vi "Stepper Sequence.vi"() -> ()   [LabVIEW 2013, in "LabVIEW Interface for Arduino.lvlib"]
doc: "Writes specified digital values to all 14 digital I/O pins. Each pin must first be configured as a digital output using the Arduino Set Digital Pin Mode VI."
uses:
  <vilib>/LabVIEW Interface for Arduino/LabVIEW Interface for Arduino.lvlib
  Hello Optotune Lens (30.06.2014)/Calibration.ctl
  <vilib>/LabVIEW Interface for Arduino/Type Defs/Board Type.ctl
  <vilib>/LabVIEW Interface for Arduino/Type Defs/Analog Pin.ctl
  <vilib>/Instr/_visa.llb/VISA Configure Serial Port (Instr).vi
panel:
  out "Array":dbl[](array[numeric])
  out "Voltage":dbl(knob) scale=0.0..5.0
  out "x*y 2":dbl
  out "x*y":dbl
  out "8bit integer":i8
  out "Schritt 7":bool=TRUE
  out "Schritt 6":bool=TRUE
  out "Schritt 5":bool=TRUE
  out "Schritt 4":bool=TRUE
  out "Schritt 3":bool=TRUE
  out "Schritt 2":bool=TRUE
  out "Schritt 1":bool=TRUE
  out "Value":u8
  out "x = y?":bool
  in  "Threshold I_Focus":dbl=0.33
  out "Nummer Aktuelle Messung":i32
  out "Position_aktuell 2":dbl
  out "Result":dbl[][](array[numeric])
  out "x+y":dbl
  in  "STOP Process":bool
  in  "STOP INTIAL":bool
  out "VISA resource name out 3":refnum<visa-resource-name>
  out "Command to Port 2":string
  out "Number of Measurements":i8
  in  "Min Focal Length 2":dbl
  in  "Max Focal Length":dbl=293.0
  out "I_0 - I_aktuell":dbl
  out "I_new":dbl(knob) scale=0.0..5.0
  out "Steps":dbl
  out "Position_aktuell":dbl
  in  "First Motor Pin":u8=3
  in  "Pin Endlagenschalter":u8=32
  out "I_0":dbl(knob) scale=0.0..5.0
  in  "Stepwidth Focalwidth lens":dbl=50.0
  in  "Calibration":T1={"Max Current A"=293.0, "Max Current B"=293.0, "UCL A"=300.0, "UCL B"=300.0, "LCL A"=0.0, "LCL B"=0.0} {"Max Current A" format="%#_g mA"; "Max Current B" format="%#_g mA"; "UCL A" format="%#_g mA"; "LCL A" format="%#_g mA"; "UCL B" format="%#_g mA"; "LCL B" format="%#_g mA"}
  out "ID":u16
  out "VISA resource name out":string
  out "Calibration 2":T1 {"Max Current A" format="%#_g mA"; "Max Current B" format="%#_g mA"; "UCL A" format="%#_g mA"; "LCL A" format="%#_g mA"; "UCL B" format="%#_g mA"; "LCL B" format="%#_g mA"}
  out "OK":bool
  out "Data":string
  out "Command to Port":string
  out "TA (°C)":dbl
  out "error out":errorcluster
  in  "error in (no error)":errorcluster
  in  "VISA resource name":string="COM13"
  in  "Initial Speed":dbl=1.0
  # "Lens Settings"
  # "Diodenstrom I0"
  # "Measurement Settings"
  # "Initial Settings"
  # "mA"
  # "0 Fast, 100 slow"
  # "mA"
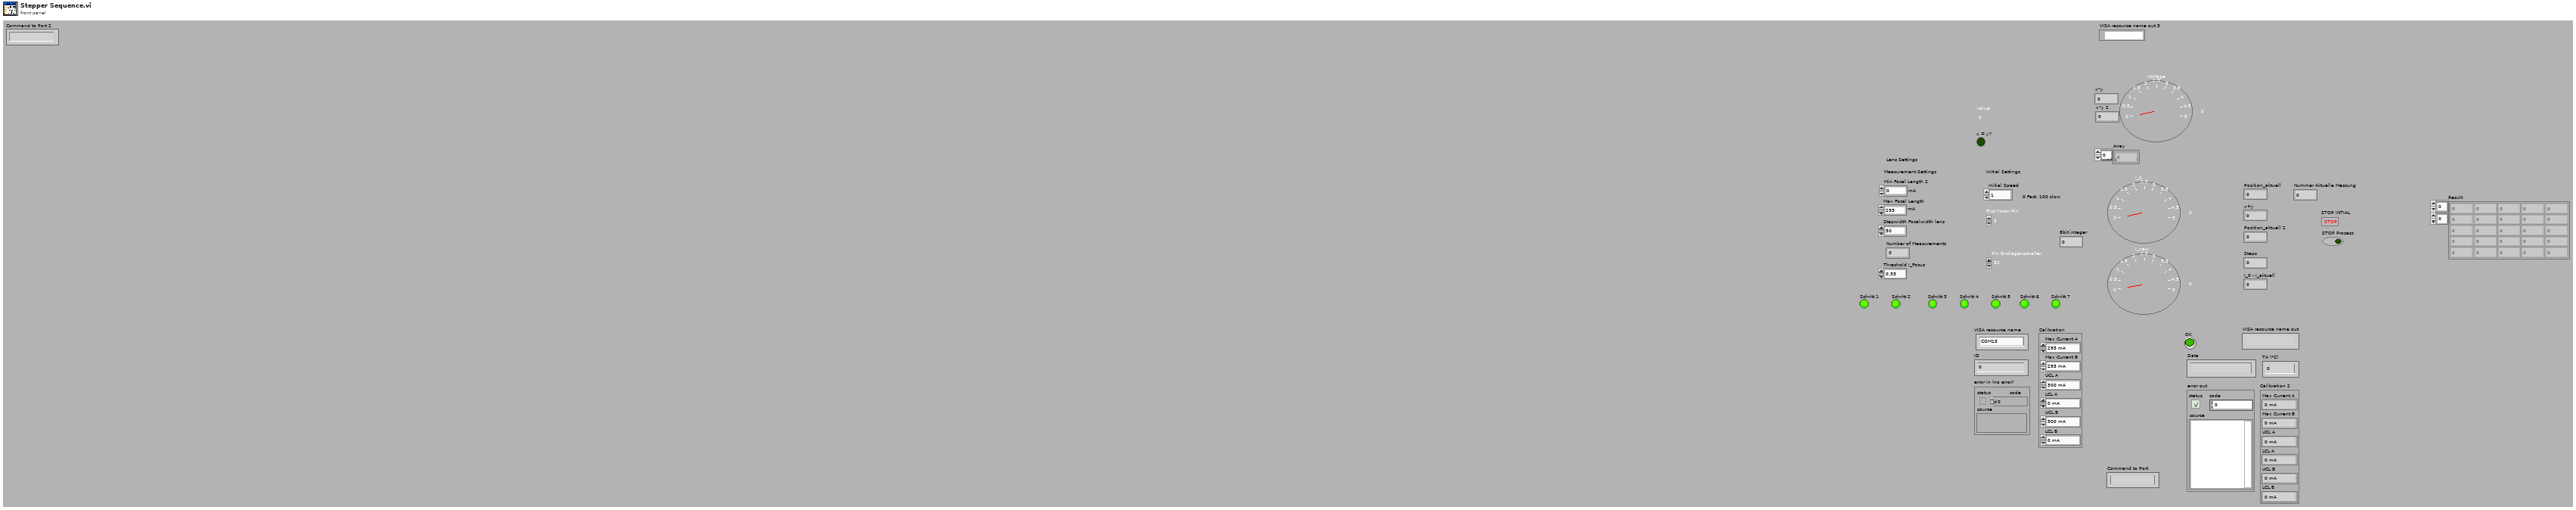
[diagram p1: front panel]
types:
  T1 = typedef "Calibration.ctl" = cluster{"Max Current A":dbl, "Max Current B":dbl, "UCL A":dbl, "UCL B":dbl, "LCL A":dbl, "LCL B":dbl}
  T2 = typedef "LabVIEW Interface for Arduino.lvlib/Board Type.ctl" = enum16{"Uno", "Dimuelanove w/Atmega 328", "Mega 2560"}
  T3 = typedef "LabVIEW Interface for Arduino.lvlib/Arduino Resource.ctl" = cluster{"VISA resource":refnum<visa-resource-name>, "Board Type":T2, "Connection Type":enum8{"USB / Serial"}, "Bytes Per Packet (15)":u8}
  T4 = typedef "LabVIEW Interface for Arduino.lvlib/Analog Pin.ctl" = enum8{"Anlog In 0", "Anlog In 1", "Anlog In 2", "Anlog In 3", "Anlog In 4", "Anlog In 5"}
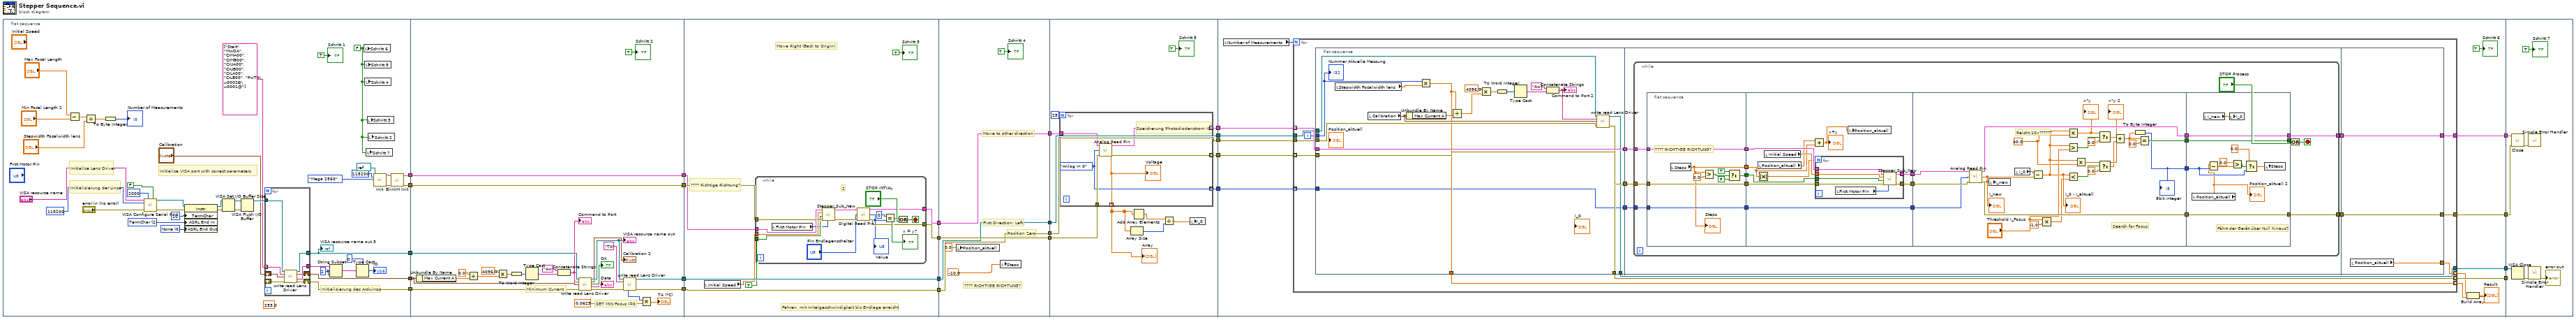
[diagram p0: block diagram]
diagram:
  n1 = flat-sequence {
    tunnel: [w44] -> w16
    tunnel: [w43] -> w15
    tunnel: [w42] -> w14
    tunnel: [w37] -> w3
    tunnel: [w36] -> w2
    tunnel: [w78] -> w26
    tunnel: [w77] -> w25
    tunnel: w16 -> [w100]
    tunnel: w15 -> [w99]
    tunnel: w14 -> [w98]
    tunnel: [w95] -> w13
    tunnel: [w79] -> w4
    tunnel: w3 -> [w78]
    tunnel: w2 -> [w77]
    tunnel: [w108] -> w20
    tunnel: w26 -> [w106]
    tunnel: [w107] -> w18
    tunnel: w25 -> [w109]
    tunnel: w13 -> [w105]
    tunnel: [w105] -> w12
    tunnel: [w104] -> w5
    tunnel: w4 -> [w104]
    tunnel: w20 -> [w131]
    tunnel: [w131] -> w19
    tunnel: w18 -> [w130]
    tunnel: [w130] -> w17
    tunnel: w12 -> [w129]
    tunnel: [w129] -> w11
    tunnel: [w128] -> w6
    tunnel: w5 -> [w128]
    tunnel: w19 -> [w143]
    tunnel: [w142] -> w24
    tunnel: w17 -> [w144]
    tunnel: [w141] -> w23
    tunnel: w11 -> [w140]
    tunnel: [w140] -> w10
    tunnel: [w139] -> w7
    tunnel: w6 -> [w139]
    tunnel: [w138] -> w1
    tunnel: w24 -> [w164]
    tunnel: w23 -> [w163]
    tunnel: [w162] -> w22
    tunnel: [w161] -> w21
    tunnel: w10 -> [w158]
    tunnel: [w159] -> w9
    tunnel: [w157] -> w8
    tunnel: w7 -> [w156]
    tunnel: w1 -> [w152]
    tunnel: w22 -> [w293]
    tunnel: w21 -> [w292]
    tunnel: w9 -> [w294]
    tunnel: w8 -> [_]
    frame #0 {
      w28 = FALSE ("Schritt 6")
      (unwired) 293.0
      w64 = 2 ("length (rest)")
      w49 = u16 0 items=["None", "Last Bit", "TermChar", "Break"] ("Serial Settings:End Mode for Writes")
      w50 = u16 2 items=["None", "Last Bit", "TermChar"] ("Serial Settings:End Mode for Reads")
      # "Initialisierung des Arduinos"
      # "Initialisierung der Linse"
      # "Initialize Lens Driver"
      # "Initialize VISA port with correct parameters"
      n2 = Subtract(x="Max Focal Length", y="Min Focal Length 2") -> (x-y=w33:dbl)
      n3 = Divide(x=w33, y="Stepwidth Focalwidth lens") -> (x/y=w31:dbl)
      n4 = To Byte Integer(number=w31) -> (8bit integer=→"Number of Measurements":i8)
      n5 = call-poly "VISA Configure Serial Port"("VISA resource name"="VISA resource name", "timeout (10sec)"=u32 2000, "Enable Termination\nChar (T)"=FALSE ("Enable Termination\nChar (T)"), "baud rate (9600)"=u32 115200, "error in (no error)"="error in (no error)") -> ("VISA resource name out"=w54:refnum<visa-resource-name>, "error out"=w52:errorcluster)  [unwired: 9 in]
      n6 = property class="Instr"(reference=w54, error in=w52, "TermChar"=u8 10 ("Message Based Settings:Termination Character"), "ASRL End In"=w50, "ASRL End Out"=w49) -> (reference out=w53:refnum<visa-resource-name>, error out=w51:errorcluster)
      n7 = VISA Set I/O Buffer Size(VISA resource name=w53, error in (no error)=w51) -> (VISA resource name out=w46:refnum<visa-resource-name>, error out=w45:errorcluster)  [unwired: 2 in]
      n8 = VISA Flush I/O Buffer(VISA resource name=w46, error in (no error)=w45) -> (VISA resource name out=w66:refnum<visa-resource-name>)  [unwired: 1 in, 1 out]
      n9 = for {
        tunnel: w66 -> [w73]
        tunnel: [w70] -> w44
        tunnel: string[] ["Start", "MwDA", "CrMA00", "CrMB00", "CrUA00", "CrUB00", "CrLA00", "CrLB00", "PwTA\u0002Ð\u0001@"] -> [w68] mode=indexing
        tunnel: [w67] -> w60
        shift-right: [w71] -> w43
        shift-left: "Calibration" -> [w72]
        shift-right: [w69] -> w42
        shift-left: _ -> [w74]
        n10 = call "write read Lens Driver.vi"("VISA resource name"=w73, "command"=w68, "Calibration"=w72, "error in (no error)"=w74) -> ("VISA resource name out"=w70:refnum<visa-resource-name>, "Calibration 2"=w71:T1, "Data"=w67:string, "error out"=w69:errorcluster)  [unwired: 4 in, 4 out]
      }
      "VISA resource name out 3" <- w44
      n11 = String Subset(string=w60, offset (0)=w64, length (rest)=w64) -> (substring=w62:string)
      n12 = Type Cast(type=u16 0 ("length (rest)"), x=w62) -> (*(type *) &x=→"ID":u16)
      n13 = local write "Schritt 6"(w28) -> ()
      n14 = local write "Schritt 5"(w28) -> ()
      n15 = local write "Schritt 4"(w28) -> ()
      n16 = local write "Schritt 7"(w28) -> ()
      n17 = local write "Schritt 3"(w28) -> ()
      n18 = local write "Schritt 2"(w28) -> ()
      n19 = call <vilib>:"Init.vi"("VISA resource"=refnum<visa-resource-name> refnum, "Baud Rate (115200)"=u32 115200, "Board Type (Uno)"=Board_Type."Mega 2560") -> ("Arduino Resource"=w40:T3, "error out"=w41:errorcluster)  [unwired: 15 in]
      n20 = call <vilib>:"BlinkM Init.vi"("Arduino Resource"=w40, "error in"=w41) -> ("Arduino Resource"=w37:T3, "error out"=w36:errorcluster)  [unwired: 12 in]
      "Schritt 1" <- TRUE
    }
    frame #1 {
      # "Minimum Current"
      # "SET MIN Focus I=0"
      n21 = Unbundle By Name(w99) -> ("Max Current A"=w84:dbl)
      n22 = Divide(x=0.0, y=w84) -> (x/y=w91:dbl)
      n23 = Multiply(x=4096.0, y=w91) -> (x*y=w89:dbl)
      n24 = To Word Integer(number=w89) -> (16bit integer=w88:i16)
      n25 = Type Cast(x=w88) -> (*(type *) &x=w87:string)  [unwired: 1 in]
      n26 = Concatenate Strings("Aw", w87) -> (w85:string)
      "Command to Port" <- w85
      n27 = call "write read Lens Driver.vi"("VISA resource name"=w100, "command"=w85, "Calibration"=w99, "error in (no error)"=w98) -> ("VISA resource name out"=w97:refnum<visa-resource-name>, "Calibration 2"=→"Calibration 2":T1, "OK"=→"OK":bool, "Data"=→"Data":string, "error out"=w96:errorcluster)  [unwired: 4 in, 3 out]
      "VISA resource name out" <- w97
      n28 = call "write read Lens Driver.vi"("VISA resource name"=w97, "command"="TA", "error in (no error)"=w96) -> ("VISA resource name out"=w95:refnum<visa-resource-name>, "TA"=w81:u16, "error out"=w79:errorcluster)  [unwired: 5 in, 5 out]
      n29 = Multiply(x=w81, y=0.0625) -> (x*y=→"TA (°C)":dbl)
      "Schritt 2" <- TRUE
    }
    frame #2 {
      # "???? Richtige Richtung?"
      # "Move Right (Back to Origin)"
      # "Fahren, mit Initalgeschwindigkeit bis Endlage erreicht"
      n30 = local read "Initial Speed"() -> (w103:dbl)
      n31 = while {
        tunnel: w106 -> [w123]
        tunnel: w109 -> [w122]
        tunnel: TRUE -> [w120]
        tunnel: w103 -> [w121]
        tunnel: [w115] -> w108
        tunnel: [w114] -> w107
        stop <- w117 stop-if-true
        # "2"
        n32 = local read "First Motor Pin"() -> (w119:u8)
        n33 = call "Stepper_Sub_New.vi"("First Motor Pin"=w119, "error in"=w122, "Direction"=w120, "Velocity"=w121, "Arduino Resource"=w123) -> ("error out"=w112:errorcluster, "Arduino Resource 2"=w111:T3)  [unwired: 5 in]
        n34 = call <vilib>:"Digital Read Pin.vi"("Arduino Resource"=w111, "Digital I/O Pin (0)"="Pin Endlagenschalter", "error in"=w112) -> ("Arduino Resource"=w115:T3, "Value"=w113:u8, "error out"=w114:errorcluster)  [unwired: 10 in]
        "Value" <- w113
        n35 = Equal?(x=u8 0, y=w113) -> (x = y?=w118:bool)
        "x = y?" <- w118
        n36 = Or(x=w118, y="STOP INTIAL") -> (x .or. y?=w117:bool)
      }
      "Schritt 3" <- TRUE
    }
    frame #3 {
      # "???? RICHTIGE RICHTUNG?"
      # "Move to other direction"
      # "First Direction: Left"
      # "Position Zero"
      n37 = local write "Position_aktuell"(0.0 ("Position_aktuell")) -> ()
      n38 = local write "Steps"(-10.0 ("Position_aktuell")) -> ()
      "Schritt 4" <- TRUE
    }
    frame #4 {
      n39 = for {
        N: 25 -> [_]
        tunnel: w144 -> [w150]
        tunnel: w143 -> [w149]
        tunnel: [w148] -> w142 mode=indexing
        tunnel: [w147] -> w141 mode=indexing
        tunnel: [w146] -> w138 mode=indexing
        tunnel: [w145] -> w136 mode=indexing
        w146 = Analog_Pin."Anlog In 0" ("Photodiode Pin")
        # "Speicherung Photodiodenstrom I0"
        n40 = call <vilib>:"Analog Read Pin.vi"("Arduino Resource"=w149, "Analog Input Pin (0)"=w146, "error in"=w150) -> ("Arduino Resource"=w148:T3, "Voltage"=w145:dbl, "error out"=w147:errorcluster)  [unwired: 10 in]
        "Voltage" <- w145
      }
      "Array" <- w136
      n41 = Array Size(array=w136) -> (size(s)=w134:i32)
      n42 = Add Array Elements(numeric array=w136) -> (sum=w135:dbl)
      n43 = Divide(x=w135, y=w134) -> (x/y=w133:dbl)
      n44 = local write "I_0"(w133) -> ()
      "Schritt 5" <- TRUE
    }
    frame #5 {
      n45 = local read "Number of Measurements"() -> (w160:i8)
      n46 = for {
        N: w160 -> [_]
        tunnel: w164 -> [w181] mode=indexing
        tunnel: w163 -> [w180] mode=indexing
        tunnel: [w179] -> w162
        tunnel: [w178] -> w161
        tunnel: w158 -> [w175]
        tunnel: w156 -> [w174]
        tunnel: [w172] -> w159
        tunnel: [w171] -> w157 mode=indexing
        tunnel: [w168] -> w155 mode=indexing
        tunnel: [w167] -> w154 mode=indexing
        tunnel: w152 -> [w165] mode=indexing
        i -> [w173]
        n47 = flat-sequence {
          tunnel: w181 -> [w200]
          tunnel: [w200] -> w177
          tunnel: w180 -> [w199]
          tunnel: [w199] -> w176
          tunnel: w175 -> [w191]
          tunnel: w174 -> [w190]
          tunnel: w173 -> [w187]
          tunnel: [w186] -> w172
          tunnel: [w185] -> w171
          tunnel: [w183] -> w167
          tunnel: [w182] -> w166
          tunnel: w165 -> [w182]
          tunnel: w177 -> [w205]
          tunnel: w176 -> [w204]
          tunnel: [w203] -> w170
          tunnel: [w202] -> w169
          tunnel: w166 -> [w201]
          tunnel: [w289] -> w178
          tunnel: [w290] -> w179
          tunnel: w170 -> [w290]
          tunnel: w169 -> [w289]
          tunnel: [w288] -> w168
          frame #0 {
            n48 = local read "Stepwidth Focalwidth lens"() -> (w188:dbl)
            n49 = local read "Calibration"() -> (w184:T1)
            n50 = Unbundle By Name(w184) -> ("Max Current A"=w189:dbl)
            n51 = Multiply(x=w187, y=w188) -> (x*y=w183:dbl)
            n52 = Divide(x=w183, y=w189) -> (x/y=w198:dbl)
            n53 = Multiply(x=4096.0, y=w198) -> (x*y=w196:dbl)
            n54 = To Word Integer(number=w196) -> (16bit integer=w195:i16)
            n55 = Type Cast(x=w195) -> (*(type *) &x=w194:string)  [unwired: 1 in]
            n56 = Concatenate Strings("Aw", w194) -> (w192:string)
            "Command to Port 2" <- w192
            n57 = call "write read Lens Driver.vi"("VISA resource name"=w191, "command"=w192, "Calibration"=w184, "error in (no error)"=w190) -> ("VISA resource name out"=w186:refnum<visa-resource-name>, "error out"=w185:errorcluster)  [unwired: 4 in, 6 out]
            "Nummer Aktuelle Messung" <- w187
          }
          frame #1 {
            n58 = while {
              tunnel: w205 -> [w223]
              tunnel: w204 -> [w222]
              tunnel: [w221] -> w203
              tunnel: [w220] -> w202
              tunnel: w201 -> [w207]
              stop <- w218 stop-if-true
              n59 = flat-sequence {
                tunnel: w222 -> [w233]
                tunnel: w223 -> [w234]
                tunnel: [w234] -> w214
                tunnel: [w233] -> w213
                tunnel: [w226] -> w212
                tunnel: [w228] -> w211
                tunnel: [w227] -> w208
                tunnel: w207 -> [w227]
                tunnel: [w243] -> w224
                tunnel: [w242] -> w225
                tunnel: w214 -> [w245]
                tunnel: w213 -> [w244]
                tunnel: w212 -> [w238]
                tunnel: w211 -> [w240]
                tunnel: [w235] -> w209
                tunnel: w208 -> [w235]
                tunnel: w225 -> [w273]
                tunnel: w224 -> [w274]
                tunnel: [w276] -> w217
                tunnel: [w275] -> w216
                tunnel: [w259] -> w215
                tunnel: w209 -> [w255]
                tunnel: [w254] -> w206
                tunnel: [w285] -> w219
                tunnel: [w286] -> w220
                tunnel: [w287] -> w221
                tunnel: w217 -> [w287]
                tunnel: w216 -> [w286]
                tunnel: w215 -> [w285]
                tunnel: w206 -> [w279]
                frame #0 {
                  # "???? RICHTIGE RICHTUNG?"
                  n60 = local read "Steps"() -> (w226:dbl)
                  "Steps" <- w226
                  n61 = Greater?(x=w226, y=0.0) -> (0:w231:bool)
                  n62 = Select(t=TRUE, s=w231, f=FALSE) -> (s? t:f=w228:bool)
                }
                frame #1 {
                  n63 = Absolute Value(x=w238) -> (abs(x)=w236:dbl)
                  n64 = local read "Position_aktuell"() -> (w239:dbl)
                  n65 = local read "Initial Speed"() -> (w241:dbl)
                  n66 = Add(x=w239, y=w238) -> (x+y=w237:dbl)
                  "x+y" <- w237
                  n67 = for {
                    N: w236 -> [_]
                    tunnel: w245 -> [w252]
                    tunnel: w244 -> [w251]
                    tunnel: [w247] -> w243
                    tunnel: [w246] -> w242
                    tunnel: w241 -> [w250]
                    tunnel: w240 -> [w249]
                    n68 = local read "First Motor Pin"() -> (w248:u8)
                    n69 = call "Stepper_Sub_New.vi"("First Motor Pin"=w248, "error in"=w251, "Direction"=w249, "Velocity"=w250, "Arduino Resource"=w252) -> ("error out"=w246:errorcluster, "Arduino Resource 2"=w247:T3)  [unwired: 5 in]
                  }
                  n70 = local write "Position_aktuell"(w237) -> ()
                }
                frame #2 {
                  w253 = 40.0 ("x")
                  # "Reicht 10x??????"
                  # "Search for Focus"
                  n71 = call <vilib>:"Analog Read Pin.vi"("Arduino Resource"=w274, "Analog Input Pin (0)"=w255, "error in"=w273) -> ("Arduino Resource"=w276:T3, "Voltage"=w272:dbl, "error out"=w275:errorcluster)  [unwired: 10 in]
                  "I_new" <- w272
                  n72 = local write "I_new"(w272) -> ()
                  n73 = local read "I_0"() -> (w271:dbl)
                  n74 = Subtract(x=w271, y=w272) -> (x-y=w265:dbl)
                  "I_0 - I_aktuell" <- w265
                  n75 = Multiply(x="Threshold I_Focus", y=-1.0) -> (x*y=w257:dbl)
                  n76 = Multiply(x=w253, y=w265) -> (x*y=w269:dbl)
                  "x*y" <- w269
                  n77 = Greater?(x=w265, y="Threshold I_Focus") -> (0:w270:bool)
                  n78 = Less?(x=w265, y=w257) -> (x < y?=w264:bool)
                  n79 = Multiply(x=w265, y=w253) -> (x*y=w267:dbl)
                  "x*y 2" <- w267
                  n80 = Select(t=w269, s=w270, f=0.0) -> (s? t:f=w263:dbl)
                  n81 = Select(t=w267, s=w264, f=0.0) -> (s? t:f=w262:dbl)
                  n82 = Add(x=w263, y=w262) -> (x+y=w261:dbl)
                  n83 = To Byte Integer(number=w261) -> (8bit integer=w254:i8)
                  "8bit integer" <- w254
                  n84 = Equal?(x=w261, y=0.0) -> (x = y?=w259:bool)
                }
                frame #3 {
                  # "Fährt der Gerät über Null hinaus?"
                  n85 = local read "Position_aktuell"() -> (w277:dbl)
                  "Position_aktuell 2" <- w277
                  n86 = local read "I_new"() -> (w284:dbl)
                  n87 = Subtract(x=w277, y=w279) -> (x-y=w283:dbl)
                  n88 = local write "I_0"(w284) -> ()
                  n89 = Greater?(x=0.0, y=w283) -> (0:w281:bool)
                  n90 = Select(t=0.0, s=w281, f=w279) -> (s? t:f=w278:dbl)
                  n91 = local write "Steps"(w278) -> ()
                }
              }
              n92 = Or(x=w219, y="STOP Process") -> (x .or. y?=w218:bool)
            }
          }
          frame #2 {
            n93 = local read "Position_aktuell"() -> (w288:dbl)
          }
        }
      }
      n94 = Build Array(w155, w154) -> (→"Result":dbl[][])
      "Schritt 6" <- TRUE
    }
    frame #6 {
      n95 = call <vilib>:"Close.vi"("Arduino Resource"=w293, "error in"=w292) -> ("error out"=w297:errorcluster)  [unwired: 13 in]
      n96 = VISA Close(VISA resource name=w294) -> (error out=w295:errorcluster)  [unwired: 1 in]
      n97 = call <vilib>:"Simple Error Handler.vi"("error in (no error)"=w297) -> ()  [unwired: 4 in, 5 out]
      n98 = call <vilib>:"Simple Error Handler.vi"("error in (no error)"=w295) -> ("error out"=→"error out":errorcluster)  [unwired: 4 in, 4 out]
      "Schritt 7" <- TRUE
    }
  }
